vi "Write Header - CCD operation Mode.vi"(8 "error in (no error)":errorcluster, 11 "Save Image in":refnum<class "Save Image.lvclass">) -> (0 "error out":errorcluster, 3 "Save Image out":refnum<class "Save Image.lvclass">)   [LabVIEW 2018, in "Save Image.lvclass"]
uses:
  Save Image.lvclass
  <userlib>/atmcd32d.llb/Shutter_mode typedef.ctl
  <userlib>/atmcd32d.llb/ReadMode_mode typedef.ctl
  <userlib>/atmcd32d.llb/AcquisitionMode_mode typedef.ctl
  Save Image.lvclass/Save Image.ctl
  Interface/Interface.lvclass/Interface.ctl
  Simulated_Header/write keyword - integer.vi
  Simulated_Header/write keyword - string.vi
  Simulated_Header/write keyword - float.vi
  Simulated_Header/write keyword - boolean.vi
  Interface/Interface.lvclass
  <vilib>/Utility/Data Type/NI_Data Type.lvlib
  Simulated_Header/Simulated_Header.lvclass
panel:
  out "Previous SET parameters":T1
  out "CCD Config":T5
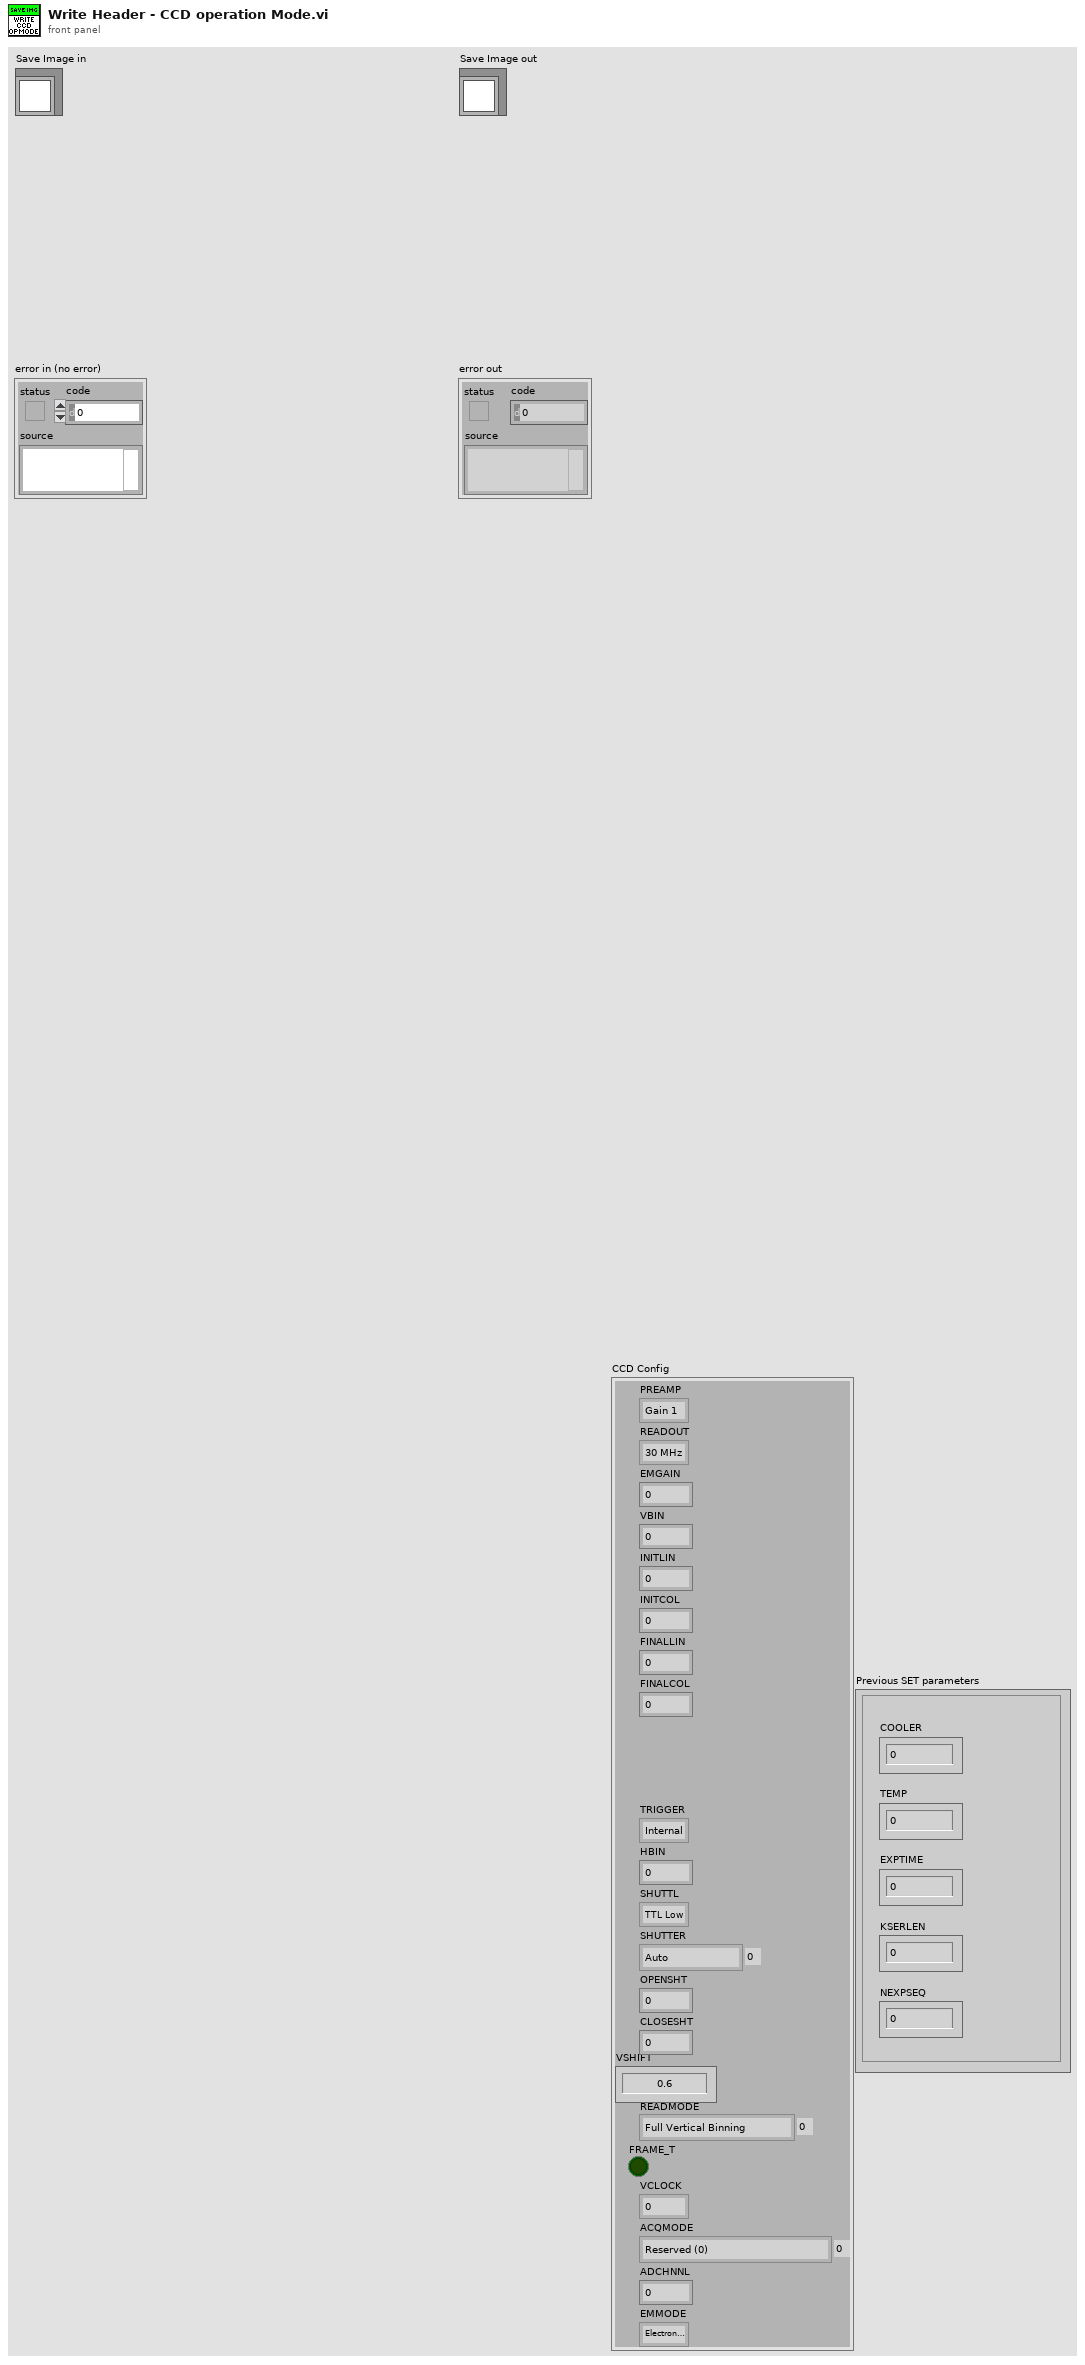
[diagram p1: front panel]
types:
  T1 = cluster{"COOLER":u16, "TEMP":i32, "EXPTIME":dbl, "KSERLEN":u32, "NEXPSEQ":u32}
  T2 = typedef "Shutter_mode typedef.ctl" = enum16{"Auto", "Open", "Close", "N/A (3)", "Open FVB Series", "Open Any Series"}
  T3 = typedef "ReadMode_mode typedef.ctl" = enum16{"Full Vertical Binning", "Multi-Track", "Random-Track", "Single-Track", "Image"}
  T4 = typedef "AcquisitionMode_mode typedef.ctl" = enum16{"Reserved (0)", "Single Scan", "Accumulate", "Kinetics", "Fast Kinetics", "Run Till Abort", "Reserved (6)", "Reserved (7)", "Reserved (8)", "Time Delayed Integration"}
  T5 = cluster{"PREAMP":enum16{"Gain 1", "Gain 2"}, "READOUT":enum16{"30 MHz", "20 MHz", "10 MHz", "1 MHz", "0.1 MHz"}, "EMGAIN":u16, "VBIN":u16, "INITLIN":u16, "INITCOL":u16, "FINALLIN":u16, "FINALCOL":u16, "TRIGGER":enum16{"Internal", "External", "N/A", "N/A_1", "N/A_2", "N/A_3", "External Start"}, "HBIN":u16, "SHUTTL":enum16{"TTL Low", "TTL High"}, "SHUTTER":T2, "OPENSHT":u16, "CLOSESHT":u16, "VSHIFT":enum16{"0.6", "1.13", "2.2", "4.33"}, "READMODE":T3, "FRAME_T":bool, "VCLOCK":enum16{"0", "+1", "+2", "+3", "+4"}, "ACQMODE":T4, "ADCHNNL":u16, "EMMODE":enum16{"Electron Multiplying", "Conventional"}}
  T6 = cluster{"PREAMP":u16, "READOUT_RATE":u16, "EM_GAIN":u16, "VBIN":u16, "INITIAL_LINE":u16, "INITIAL_COLUMN":u16, "FINAL_LINE":u16, "FINAL_COLUMN":u16, "TRIGGER_MODE":u16, "HBIN":u16, "SHUTTER_TTL":u16, "SHUTTER_MODE":u16, "SHUTTER_OPENING_TIME":u16, "SHUTTER_CLOSING_TIME":u16, "VERTICAL_SHIFT_SPEED":u16, "READ_MODE":u16, "FRAME_TRANSFER":bool, "VERTICAL_CLOCK_VOLTAGE":u16, "ACQUISITION_MODE":u16, "AD_CHANNEL":u16, "EM_MODE":u16}
  T7 = cluster{"COOLER_POWER_STATUS":u16, "TEMP":i32, "EXPTIME":dbl, "#FRAMES":u32, "#CUBES":u32}
  T8 = typedef "NI_Data Type.lvlib/Data Type.ctl" = enum8{"Invalid Type", "Void", "I8", "I16", "I32", "I64", "U8", "U16", "U32", "U64", "Single Float", "Double Float", "Extended Float", "Single Complex", "Double Complex", "Extended Complex", "Enum U8", "Enum U16", "Enum U32", "Enum U64", "Single Float With Unit", "Double Float With Unit", "Extended Float With Unit", "Single Complex with Unit", "Double Complex with Unit", "Extended Complex with Unit", "Boolean", "String", "Path", "Picture", "Tag", "Array", "Cluster", "Variant", "LV Variant", "Waveform", "Timestamp", "Digital Waveform", "Digital Data", "ExpressData", "Refnum", "External Data", "VI", "Poly VI", "LabVIEW Class Instance", "Fixed Point"}
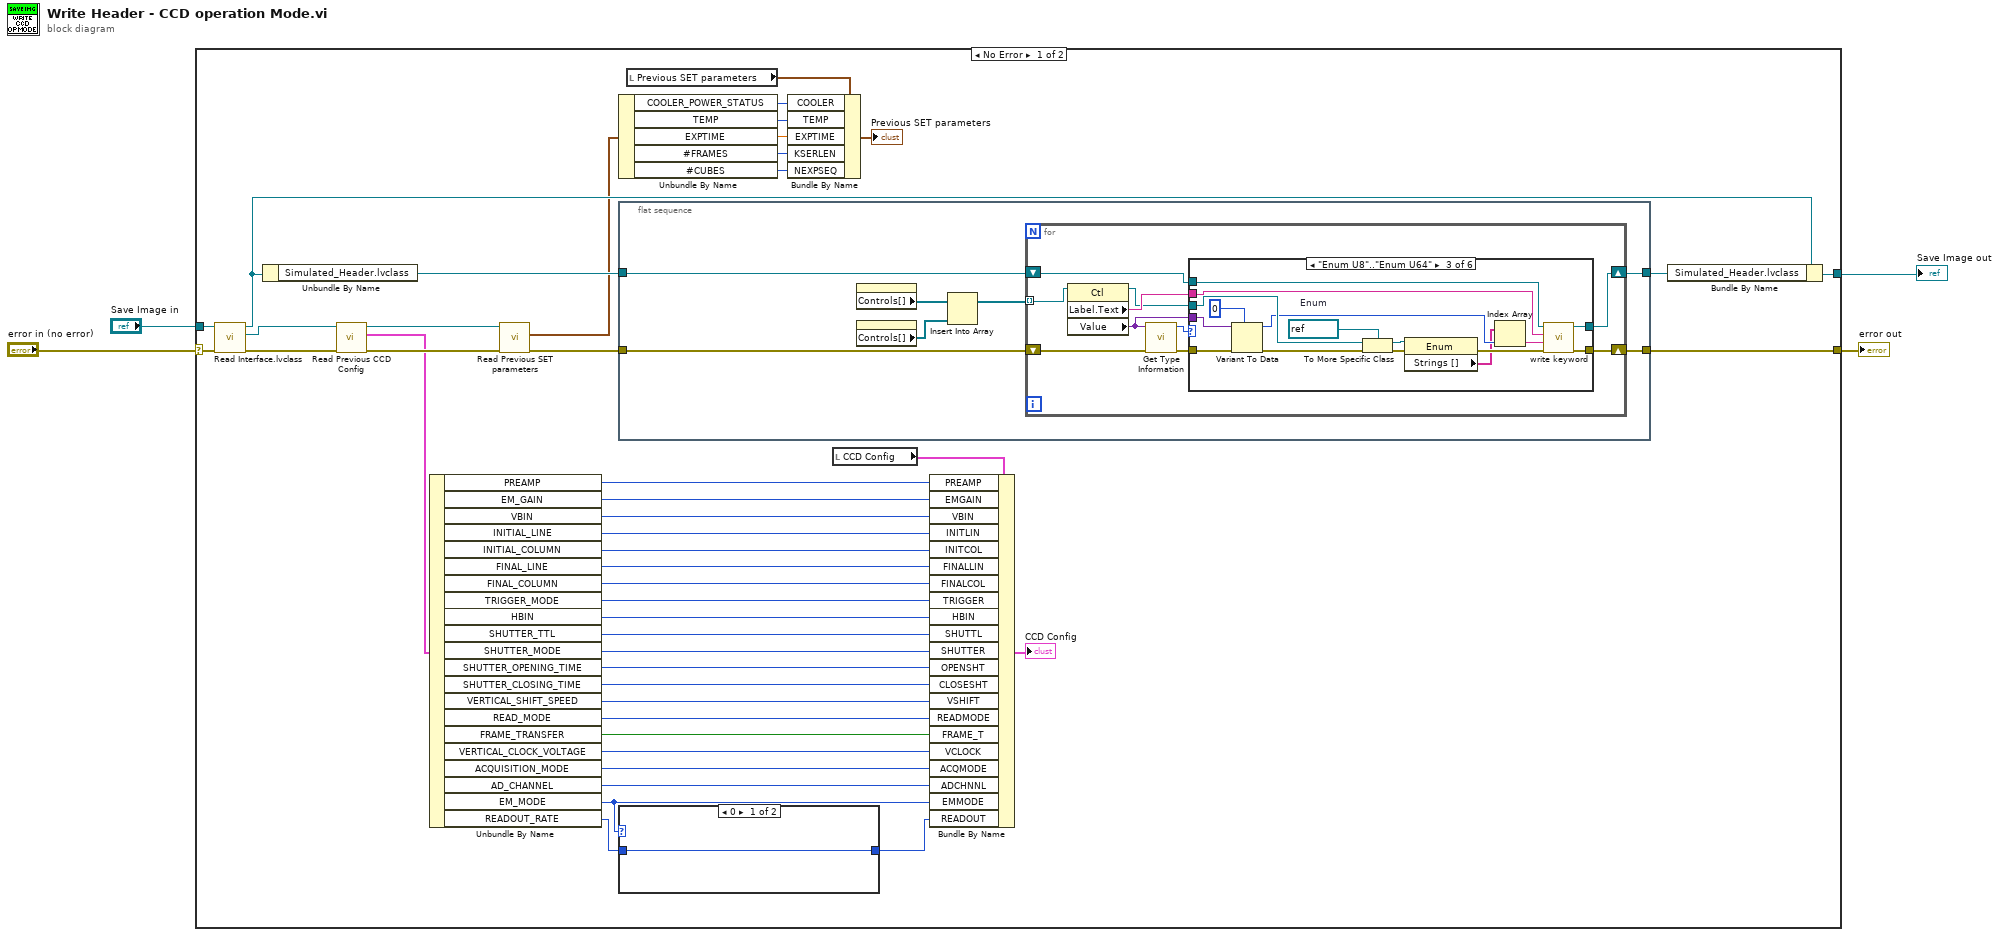
[diagram p0: block diagram]
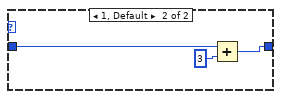
[diagram p2: hidden frame]
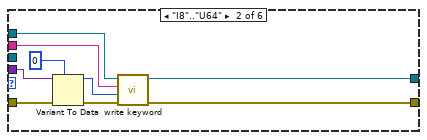
[diagram p4: hidden frame]
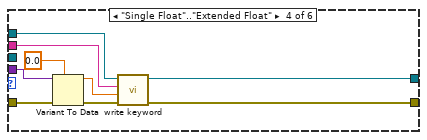
[diagram p5: hidden frame]
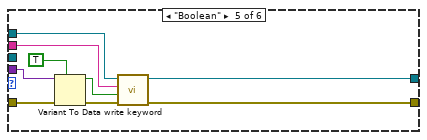
[diagram p6: hidden frame]
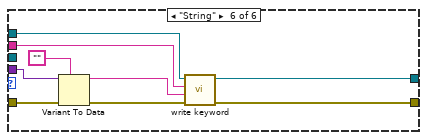
[diagram p7: hidden frame]
diagram:
  n1 = case shown="No Error" "error in (no error)" {
    selector: "error in (no error)" -> [w49 w125]
    tunnel: [w38 w125] -> w3
    tunnel: [w39 w126] -> w1
    tunnel: "Save Image in" -> [w48 w126]
    frame No Error {
      n2 = call "Read Interface.lvclass.vi"("error in (no error)"=w49, "Save Image in"=w48) -> ("error out"=w46:errorcluster, "Interface.lvclass"=w47:refnum<class "Interface.lvclass">, "Save Image out"=w45:refnum<class "Save Image.lvclass">)  [unwired: 7 in]
      n3 = Unbundle By Name(w45) -> ("Simulated_Header.lvclass"=w44:refnum<class "Simulated_Header.lvclass">)
      n4 = call "Read Previous CCD Config.vi"("error in (no error)"=w46, "Interface in"=w47) -> ("error out"=w41:errorcluster, "CCD Config"=w8:T6, "Interface out"=w42:refnum<class "Interface.lvclass">)  [unwired: 7 in]
      n5 = Unbundle By Name(w8) -> ("PREAMP"=w17:u16, "EM_GAIN"=w18:u16, "VBIN"=w19:u16, "INITIAL_LINE"=w20:u16, "INITIAL_COLUMN"=w21:u16, "FINAL_LINE"=w22:u16, "FINAL_COLUMN"=w23:u16, "TRIGGER_MODE"=w24:u16, "HBIN"=w25:u16, "SHUTTER_TTL"=w26:u16, "SHUTTER_MODE"=w27:u16, "SHUTTER_OPENING_TIME"=w28:u16, "SHUTTER_CLOSING_TIME"=w29:u16, "VERTICAL_SHIFT_SPEED"=w30:u16, "READ_MODE"=w31:u16, "FRAME_TRANSFER"=w32:bool, "VERTICAL_CLOCK_VOLTAGE"=w33:u16, "ACQUISITION_MODE"=w34:u16, "AD_CHANNEL"=w35:u16, "EM_MODE"=w7:u16, "READOUT_RATE"=w6:u16)
      n6 = call "Read Previous SET parameters.vi"("error in (no error)"=w41, "Interface in"=w42) -> ("error out"=w40:errorcluster, "Previous SET parameters"=w16:T7)  [unwired: 7 in, 1 out]
      n7 = Unbundle By Name(w16) -> ("COOLER_POWER_STATUS"=w13:u16, "TEMP"=w12:i32, "EXPTIME"=w11:dbl, "#FRAMES"=w10:u32, "#CUBES"=w9:u32)
      n8 = flat-sequence {
        tunnel: [w60] -> w38
        tunnel: w44 -> [w59]
        tunnel: [w58] -> w43
        tunnel: w40 -> [w57]
        frame #0 {
          n9 = property on="CCD Config" class="Clust (strict)"() -> ("Controls[]"=w56:refnum<vi>[])  [unwired: 2 in, 2 out]
          n10 = property on="Previous SET parameters" class="Clust (strict)"() -> ("Controls[]"=w55:refnum<vi>[])  [unwired: 2 in, 2 out]
          n11 = Insert Into Array(array=w56, new element=w55) -> (w54:refnum<vi>[])  [unwired: 1 in]
          n12 = for {
            shift-right: [w66] -> w58
            shift-left: w59 -> [w64]
            shift-right: [w67] -> w60
            shift-left: w57 -> [w70]
            tunnel: w54 -> [w63] mode=indexing
            n13 = property class="Ctl"(reference=w63) -> (reference out=w62:refnum<vi>, "Label.Text"=w68:string, "Value"=w65:variant)  [unwired: 1 in, 1 out]
            n14 = call <vilib>:"Get Type Information.vi"("error in (no error)"=w70, "Variant"=w65) -> ("error out"=w69:errorcluster, "Type"=w61:T8)  [unwired: 5 in, 3 out]
            n15 = case shown="\"Enum U8\"..\"Enum U64\"" w61 {
              tunnel: w69 -> [w72 w81 w97 w106 w115 w124]
              tunnel: w68 -> [_ w77 w95 w102 w111 w120]
              tunnel: [w72 w76 w94 w101 w110 w119] -> w67
              tunnel: [w71 w75 w93 w100 w109 w118] -> w66
              tunnel: w65 -> [_ w74 w92 w99 w108 w117]
              tunnel: w64 -> [w71 w73 w91 w98 w107 w116]
              tunnel: w62 -> [_ _ w89 _ _ _]
              frame "Invalid Type", Default {
              }
              frame "I8".."U64" {
                n16 = Variant To Data(error in=w81, type=0, Variant=w74) -> (data=w78:i32, error out=w79:errorcluster)
                n17 = call-poly "write keyword.vi"("error in (no error)"=w79, "Value"=w78, "keyword"=w77, "Simulated_Header in"=w73) -> ("error out"=w76:errorcluster, "Simulated_Header out"=w75:refnum<class "Simulated_Header.lvclass">)  [unwired: 6 in]
              }
              frame "Enum U8".."Enum U64" {
                w85 = refnum<vi> refnum  # Enum
                n18 = Variant To Data(error in=w97, type=0, Variant=w92) -> (data=w84:i32, error out=w88:errorcluster)
                n19 = To More Specific Class(target class=w85, reference=w89, error in=w88) -> (specific class reference=w87:refnum<vi>, error out=w86:errorcluster)
                n20 = property on="Property Node" class="Enum"(reference=w87, error in=w86) -> (error out=w90:errorcluster, "Strings []"=w83:string[])  [unwired: 1 out]
                n21 = Index Array(array=w83, index=w84) -> (element=w82:string)
                n22 = call-poly "write keyword.vi"("error in (no error)"=w90, "value"=w82, "keyword"=w95, "Simulated_Header in"=w91) -> ("error out"=w94:errorcluster, "Simulated_Header out"=w93:refnum<class "Simulated_Header.lvclass">)  [unwired: 6 in]
              }
              frame "Single Float".."Extended Float" {
                n23 = Variant To Data(error in=w106, type=0.0, Variant=w99) -> (data=w103:dbl, error out=w104:errorcluster)
                n24 = call-poly "write keyword.vi"("error in (no error)"=w104, "Value"=w103, "keyword"=w102, "Simulated_Header in"=w98) -> ("error out"=w101:errorcluster, "Simulated_Header out"=w100:refnum<class "Simulated_Header.lvclass">)  [unwired: 6 in]
              }
              frame "Boolean" {
                n25 = Variant To Data(error in=w115, type=TRUE, Variant=w108) -> (data=w112:bool, error out=w113:errorcluster)
                n26 = call-poly "write keyword.vi"("error in (no error)"=w113, "value"=w112, "keyword"=w111, "Simulated_Header in"=w107) -> ("error out"=w110:errorcluster, "Simulated_Header out"=w109:refnum<class "Simulated_Header.lvclass">)  [unwired: 6 in]
              }
              frame "String" {
                n27 = Variant To Data(error in=w124, type="", Variant=w117) -> (data=w121:string, error out=w122:errorcluster)
                n28 = call-poly "write keyword.vi"("error in (no error)"=w122, "value"=w121, "keyword"=w120, "Simulated_Header in"=w116) -> ("error out"=w119:errorcluster, "Simulated_Header out"=w118:refnum<class "Simulated_Header.lvclass">)  [unwired: 6 in]
              }
            }
          }
        }
      }
      n29 = case shown="0" w7 {
        tunnel: w6 -> [w50 w53]
        tunnel: [w50 w51] -> w5
        frame 0 {
        }
        frame 1, Default {
          n30 = Add(x=w53, y=u16 3) -> (x+y=w51:u16)
        }
      }
      n31 = local read "Previous SET parameters"() -> (w14:T1)
      n32 = Bundle By Name(cluster=w14, "COOLER"=w13, "TEMP"=w12, "EXPTIME"=w11, "KSERLEN"=w10, "NEXPSEQ"=w9) -> (→"Previous SET parameters":T1)
      n33 = local read "CCD Config"() -> (w36:T5)
      n34 = Bundle By Name(cluster=w36, "PREAMP"=w17, "EMGAIN"=w18, "VBIN"=w19, "INITLIN"=w20, "INITCOL"=w21, "FINALLIN"=w22, "FINALCOL"=w23, "TRIGGER"=w24, "HBIN"=w25, "SHUTTL"=w26, "SHUTTER"=w27, "OPENSHT"=w28, "CLOSESHT"=w29, "VSHIFT"=w30, "READMODE"=w31, "FRAME_T"=w32, "VCLOCK"=w33, "ACQMODE"=w34, "ADCHNNL"=w35, "EMMODE"=w7, "READOUT"=w5) -> (→"CCD Config":T5)
      n35 = Bundle By Name(cluster=w45, "Simulated_Header.lvclass"=w43) -> (w39:refnum<class "Save Image.lvclass">)
    }
    frame Error {
    }
  }
  "error out" <- w3
  "Save Image out" <- w1
